vi "GPS配置同步(子VI).vi"   [LabVIEW 2016, in "环境动力监测库.lvlib" / "NMEA.lvlib"]
uses:
  NMEA.lvlib
  <vilib>/Utility/config.llb/NI_LVConfig.lvlib
types:
  T1 = cluster{"监测项描述:输出":string, "连接方式":enum16{"串口", "TCP"}, "端口":string, "IP address:":string, "Port:":string, "站号":u64, "传感器型号":string, "波特率":u64, "data bits":u64, "停止位":u16, "奇偶校验":u16}
  T2 = typedef "NI_LVConfig.lvlib/Config Data RefNum.ctl" = refnum<k1>
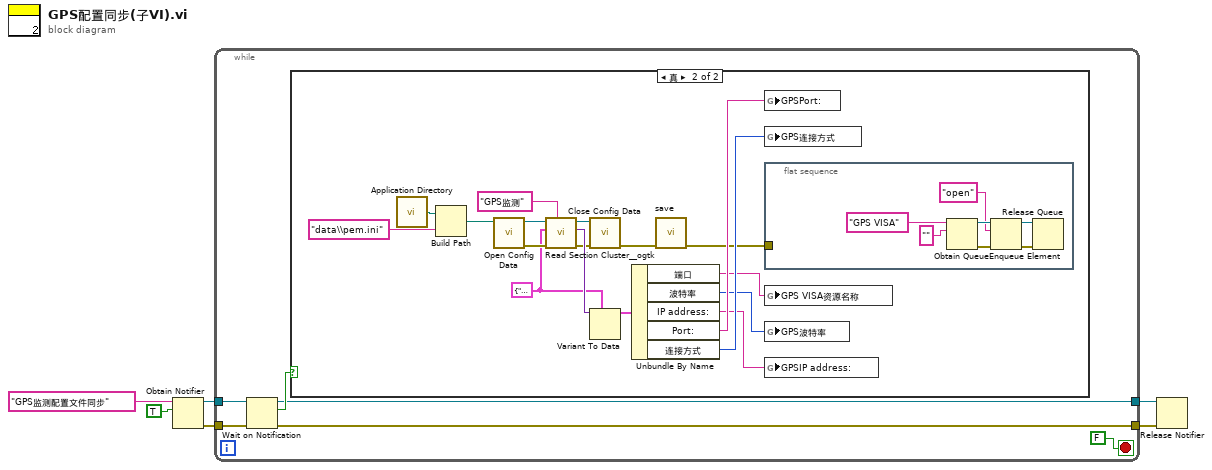
[diagram p0: block diagram]
diagram:
  n1 = Obtain Notifier(name (unnamed)="GPS监测配置文件同步" ("名称（未命名）"), notification data type=TRUE) -> (notifier out=w4:refnum<notifier>, error out=w3:errorcluster)  [unwired: 2 in, 1 out]
  n2 = while {
    tunnel: w4 -> [w12]
    tunnel: w3 -> [w11]
    tunnel: [w8] -> w2
    tunnel: [w7] -> w1
    stop <- FALSE stop-if-true
    n3 = Wait on Notification(notifier=w12, error in (no error)=w11) -> (notifier out=w8:refnum<notifier>, notification=w10:bool, error out=w7:errorcluster)  [unwired: 2 in, 1 out]
    n4 = case shown="真" w10 {
      frame False {
      }
      frame True {
        w21 = T1 {"监测项描述:输出"="", "连接方式"=enum."串口", "端口"="", "IP address:"="", "Port:"="", "站号"=19200, "传感器型号"="", "波特率"=19200, "data bits"=8, "停止位"=10, "奇偶校验"=0} ("输入簇")
        n5 = call <vilib>:"Application Directory.vi"() -> ("Application Directory"=w25:path)
        n6 = Build Path(base path=w25, name or relative path="data\\pem.ini" ("名称或相对路径")) -> (appended path=w24:path)
        n7 = call <vilib>:"Open Config Data.vi"("configuration file path"=w24) -> ("error out"=w23:errorcluster, "refnum"=w22:T2)  [unwired: 8 in, 1 out]
        n8 = call <userlib>:"Read Section Cluster__ogtk.vi"("section (optional)"="GPS监测", "error in (no error)"=w23, "Section Formatted Cluster Type"=w21, "refnum"=w22) -> ("error out"=w29:errorcluster, "Section Formatted Cluster"=w30:variant, "dup refnum"=w28:T2)  [unwired: 3 in, 2 out]
        n9 = call <vilib>:"Close Config Data.vi"("error in (no error)"=w29, "refnum"=w28) -> ("error out"=w14:errorcluster)  [unwired: 8 in, 1 out]
        n10 = Variant To Data(type=w21, Variant=w30) -> (data=w15:T1)  [unwired: 1 in, 1 out]
        n11 = Unbundle By Name(w15) -> ("端口"=w16:string, "波特率"=w17:u64, "IP address:"=w18:string, "Port:"=w19:string, "连接方式"=w20:enum16{"串口", "TCP"})
        n12 = call "save.vi"("error in (no error)"=w14) -> ("error out"=w13:errorcluster)  [unwired: 10 in]
        n13 = global write "断电保存全局变量.vi" "GPSPort:"(w19) -> ()
        n14 = global write "断电保存全局变量.vi" "GPS连接方式"(w20) -> ()
        n15 = flat-sequence {
          tunnel: w13 -> [_]
          frame #0 {
            n16 = Obtain Queue(name (unnamed)="GPS VISA" ("名称（未命名）"), element data type="") -> (queue out=w36:refnum<queue>, error out=w35:errorcluster)  [unwired: 3 in, 1 out]
            n17 = Enqueue Element(queue=w36, element="open", error in (no error)=w35) -> (queue out=w33:refnum<queue>, error out=w32:errorcluster)  [unwired: 1 in, 1 out]
            n18 = Release Queue(queue=w33, error in (no error)=w32) -> ()  [unwired: 1 in, 3 out]
          }
        }
        n19 = global write "断电保存全局变量.vi" "GPS VISA资源名称"(w16) -> ()
        n20 = global write "断电保存全局变量.vi" "GPS波特率"(w17) -> ()
        n21 = global write "断电保存全局变量.vi" "GPSIP address:"(w18) -> ()
      }
    }
  }
  n22 = Release Notifier(notifier=w2, error in (no error)=w1) -> ()  [unwired: 1 in, 3 out]
